vi "Set Camera Mode Vision Processing.vi"() -> (2 "camera mode vision":T1={"type"="camera_mode", "message"="vision"})   [LabVIEW 2016, in "Vision Server.lvclass"]
uses:
  Vision Server.lvclass
  typedef/Message Type.ctl
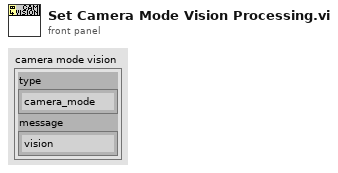
[diagram p1: front panel]
types:
  T1 = typedef "Vision Server.lvclass/Message Type.ctl" = cluster{"type":string, "message":string}
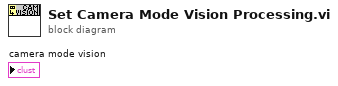
[diagram p0: block diagram]
diagram:
